vi "Manage Keyboard Events.vi"(9 "PlatMods":T1, 10 "Char":i16, 11 "Delacor_lib_QMH_Message Queue in":refnum<class "Delacor_lib_QMH_Message Queue.lvclass">) -> (0 "error out":errorcluster)   [LabVIEW 2014, in "Chart Module.lvlib"]
uses:
  Chart Module.lvlib
  <vilib>/Delacor/Delacor QMH/Libraries/Message Queue_class/Delacor_lib_QMH_Message Queue.lvclass
  <vilib>/Delacor/Delacor QMH/Libraries/Message Queue_class/Delacor_lib_QMH_Message Queue.lvclass/Delacor_lib_QMH_Message Queue.ctl
  Stop Argument--cluster.ctl
  <vilib>/Delacor/Delacor QMH/Libraries/Message Queue_class/Delacor_lib_QMH_Enqueue Message (Single).vi
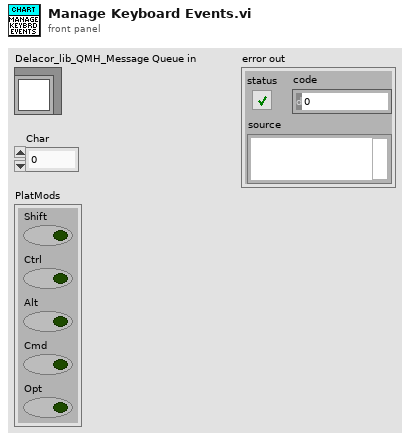
[diagram p1: front panel]
types:
  T1 = cluster{"Shift":bool, "Ctrl":bool, "Alt":bool, "Cmd":bool, "Opt":bool}
  T2 = typedef "Chart Module.lvlib/Stop Argument--cluster.ctl" = cluster{"Origin":string, "Exit via Stop Module Req?":bool}
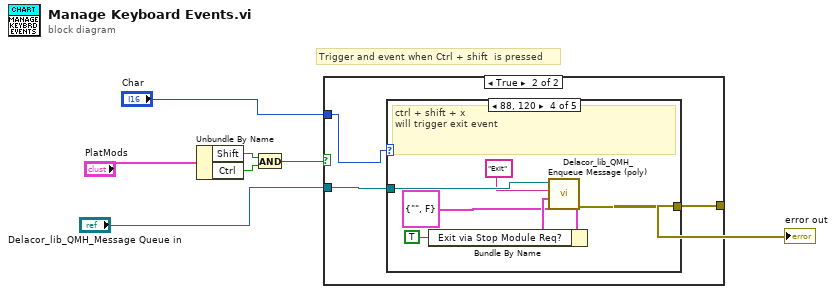
[diagram p0: block diagram]
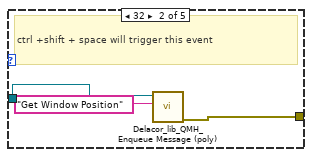
[diagram p4: hidden frame]
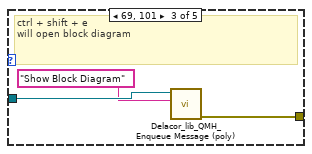
[diagram p5: hidden frame]
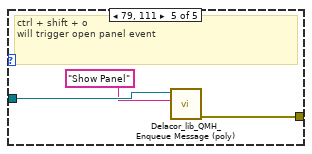
[diagram p6: hidden frame]
diagram:
  # "Trigger and event when Ctrl + shift  is pressed"
  n1 = Unbundle By Name("PlatMods") -> ("Shift"=w5:bool, "Ctrl"=w6:bool)
  n2 = And(x=w5, y=w6) -> (x .and. y?=w7:bool)
  n3 = case shown="True" w7 {
    tunnel: "Char" -> [_ w8]
    tunnel: "Delacor_lib_QMH_Message Queue in" -> [_ w10]
    tunnel: [_ w9] -> w4
    frame False {
    }
    frame True {
      n4 = case shown="88, 120" w8 {
        tunnel: w10 -> [_ w13 w15 w21 w24]
        tunnel: [_ w12 w16 w22 w25] -> w9
        frame 0, Default {
        }
        frame 32 {
          # "ctrl +shift + space will trigger this event"
          n5 = call-poly <vilib>:"Delacor_lib_QMH_Enqueue Message (poly).vi"("Message"="Get Window Position", "Message Queue in"=w13) -> ("error out"=w12:errorcluster)  [unwired: 8 in, 1 out]
        }
        frame 69, 101 {
          # "ctrl + shift + e\nwill open block diagram"
          n6 = call-poly <vilib>:"Delacor_lib_QMH_Enqueue Message (poly).vi"("Message"="Show Block Diagram", "Message Queue in"=w15) -> ("error out"=w16:errorcluster)  [unwired: 8 in, 1 out]
        }
        frame 88, 120 {
          # "ctrl + shift + x\nwill trigger exit event"
          n7 = Bundle By Name(cluster=T2 {"Origin"="", "Exit via Stop Module Req?"=FALSE} ("Stop Argument"), "Exit via Stop Module Req?"=TRUE) -> (w19:T2)
          n8 = call-poly <vilib>:"Delacor_lib_QMH_Enqueue Message (poly).vi"("Message Data"=w19, "Message"="Exit", "Message Queue in"=w21) -> ("error out"=w22:errorcluster)  [unwired: 7 in, 1 out]
        }
        frame 79, 111 {
          # "ctrl + shift + o\nwill trigger open panel event"
          n9 = call-poly <vilib>:"Delacor_lib_QMH_Enqueue Message (poly).vi"("Message"="Show Panel", "Message Queue in"=w24) -> ("error out"=w25:errorcluster)  [unwired: 8 in, 1 out]
        }
      }
    }
  }
  "error out" <- w4
